vi "ListDependencies.vi"(8 "error in (no error)":errorcluster, 11 "SMO in":refnum<class "SMO.lvclass">) -> (0 "error out":errorcluster, 1 "Level":string[](array[string]), 2 "[Dependencies]":refnum<class "SMO.lvclass">[](array[class]), 3 "SMO out":refnum<class "SMO.lvclass">)   [LabVIEW 2019, in "SMO.lvclass"]
doc: "JKI State Machine Objects (SMO) 1.3.0.56\nJKI - JKI\nCopyright (c) 2017, JKI"
uses:
  SMO.lvclass
  SMO.lvclass/SMO.ctl
  Support/Attribute.Owner/Attribute.Owner.lvclass
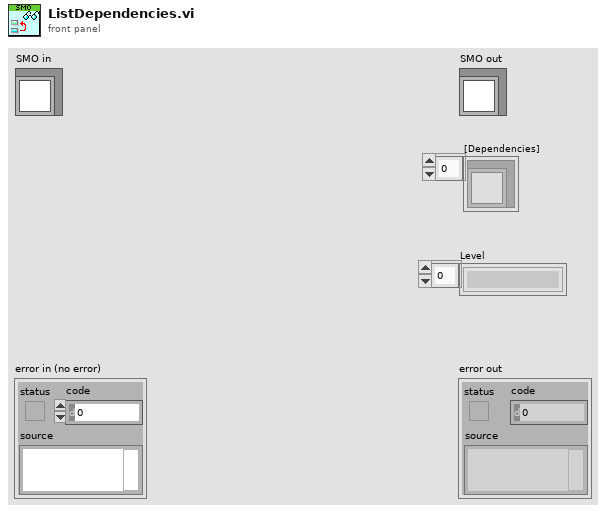
[diagram p1: front panel]
types:
  T1 = typedef "SMO.lvclass/PrivateData--Ref.ctl" = refnum<data-value>
  T2 = typedef "SMO.lvclass/PrivateData--Cluster.ctl" = cluster{"Parent Call":T3, "Registered Processes":T4[], "Sync Notifier":refnum<notifier>, "Process Error Notifier":refnum<notifier>, "Protected Events":T5, "Public Events":T6, "SMO State":T7, "[Dependencies]":T8[], "[Attributes]":refnum<class "Attribute.lvclass">[], "Launcher Close":refnum<notifier>, "Caller Watchdog":refnum<queue>, "Accessibility":T9, "NbStaticDependencies":u32}
  T3 = typedef "SMO.lvclass/Parent Call--Enum.ctl" = enum16{"Allows parent to run", "Does not request parent to run"}
  T4 = typedef "SMO.lvclass/RegisteredProcessData--Cluster.ctl" = cluster{"Name":string, "Static VI Ref":refnum<vi>, "Running":bool, "NotifierRef":u32}
  T5 = typedef "SMO.lvclass/Protected Events.ctl" = cluster{"StopProcesses":refnum<user-event>, "AbortProcesses":refnum<user-event>, "Config Changed":refnum<user-event>, "Dependency":refnum<user-event>}
  T6 = typedef "SMO.lvclass/Public Events.ctl" = cluster{"Error":refnum<user-event>, "State":refnum<user-event>, "Reserve State":refnum<user-event>}
  T7 = typedef "SMO.lvclass/SMOState --Enum.ctl" = enum16{"unknown", "Created", "Started", "Stopped"}
  T8 = typedef "SMO.lvclass/SMO Dependency--Cluster.ctl" = cluster{"Dependency":refnum<class "SMO.lvclass">, "Level":string}
  T9 = typedef "SMO.lvclass/Accessibility--Cluster.ctl" = cluster{"Lock Key":string, "Reserve State":T10}
  T10 = typedef "SMO.lvclass/Reserve State--Enum.ctl" = enum16{"Unreserved", "Reserved", "Self-locked"}
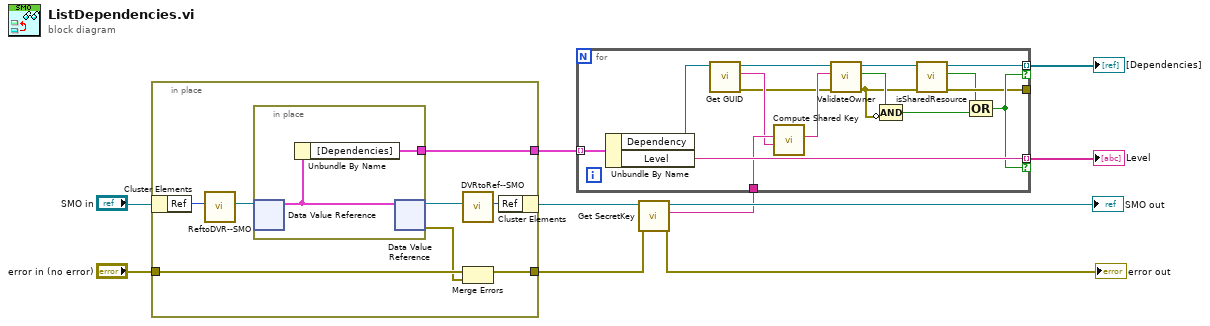
[diagram p0: block diagram]
diagram:
  n1 = in-place {
    in-place-border: "error in (no error)" -> [w14]
    in-place-border: [w12] -> w1
    in-place-border: [w11] -> w9
    n2 = in-place-cluster #1("SMO in") -> ("Ref"=w18:u32)
    n3 = call "ReftoDVR--SMO.vi"("Ref"=w18) -> ("Ref"=w17:T1)  [unwired: 10 in]
    n4 = in-place {
      in-place-border: [w19] -> w11
      n5 = in-place-dvr #2(w17) -> (w20:T2)  [unwired: 1 out]
      n6 = Unbundle By Name(w20) -> ("[Dependencies]"=w19:T8[])
      n7 = in-place-dvr #2(w20) -> (w16:T1, w13:errorcluster)
    }
    n8 = call "DVRtoRef--SMO.vi"("Ref"=w16) -> ("Ref"=w15:u32)  [unwired: 10 in]
    n9 = Merge Errors(w14, w13) -> (w12:errorcluster)
    n10 = in-place-cluster #1("Ref"=w15) -> (w5:refnum<class "SMO.lvclass">)
  }
  n11 = call "Get SecretKey.vi"("error in (no error)"=w1, "SMO"=w5) -> ("error out"=→"error out":errorcluster, "SecretKey"=w3:string, "SMO out"=→"SMO out":refnum<class "SMO.lvclass">)  [unwired: 7 in]
  n12 = for {
    tunnel: w9 -> [w36] mode=indexing
    tunnel: [w25] -> w8 mode=indexing if=w27
    tunnel: [w35] -> w7 mode=indexing if=w27
    tunnel: w3 -> [w33]
    tunnel: [w22] -> _
    n13 = Unbundle By Name(w36) -> ("Dependency"=w30:refnum<class "SMO.lvclass">, "Level"=w35:string)
    n14 = call "Get GUID.vi"("SMO"=w30) -> ("error out"=w29:errorcluster, "GUID"=w31:string, "SMO out"=w32:refnum<class "SMO.lvclass">)  [unwired: 8 in]
    n15 = call "Compute Shared Key.vi"("GUID"=w31, "SecretKey"=w33) -> ("Shared Key"=w34:string)  [unwired: 9 in]
    n16 = call "ValidateOwner.vi"("error in (no error)"=w29, "Shared Key"=w34, "SMO in"=w32) -> ("error out"=w23:errorcluster, "key matched"=w28:bool, "SMO out"=w26:refnum<class "SMO.lvclass">)  [unwired: 5 in, 1 out]
    n17 = Compound Arithmetic op=AND(w28, invert w23) -> (w24:bool)
    n18 = call "isSharedResource.vi"("error in (no error)"=w23, "SMO in"=w26) -> ("error out"=w22:errorcluster, "shared resource"=w21:bool, "SMO out"=w25:refnum<class "SMO.lvclass">)  [unwired: 7 in]
    n19 = Compound Arithmetic op=OR(w21, w24) -> (w27:bool)
  }
  "[Dependencies]" <- w8
  "Level" <- w7
